vi "ABB Attendance report.vi"(10 "Report in":string) -> (2 "Report out":string)   [LabVIEW 2017]
uses:
  ABB global.vi
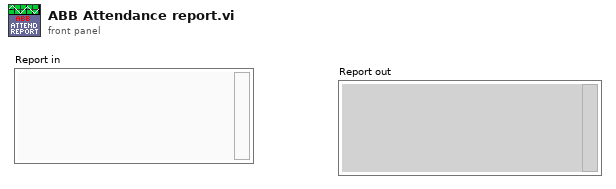
[diagram p1: front panel]
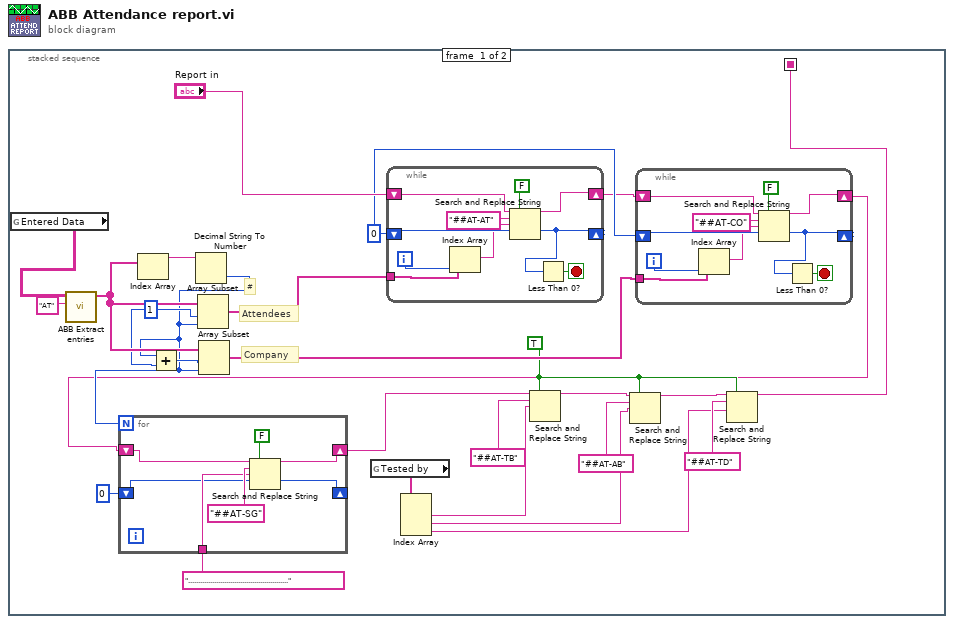
[diagram p0: block diagram]
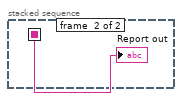
[diagram p2: hidden frame]
diagram:
  n1 = stacked-sequence {
    seq-local: [w14 _] -> [_ w55]
    frame #0 {
      w10 = TRUE ("replace all? (F)")
      w19 = 0
      w22 = 1 ("index")
      # "Company"
      # "Attendees"
      # "#"
      n2 = global read "ABB global.vi" "Entered Data"() -> (w24:string[][])
      n3 = call "ABB Extract entries.vi"("Entry ID"="AT", "Entry table in"=w24) -> ("Selected Entries"=w23:string[])  [unwired: 9 in]
      n4 = Index Array(array=w23) -> (element=w26:string)  [unwired: 1 in]
      n5 = Decimal String To Number(string=w26) -> (number=w5:i32)  [unwired: 2 in, 1 out]
      n6 = Add(x=w5, y=w22) -> (x+y=w21:i32)
      n7 = Array Subset(array=w23, index=w22, length=w5) -> (w20:string[])
      n8 = Array Subset(array=w23, index=w21, length=w5) -> (w17:string[])
      n9 = global read "ABB global.vi" "Tested by"() -> (w9:string[])
      n10 = while {
        shift-right: [w52] -> w18
        shift-left: "Report in" -> [w54]
        tunnel: w20 -> [w47]
        shift-right: [w48] -> _
        shift-left: w19 -> [w51]
        i -> [w46]
        stop <- w49 stop-if-true
        n11 = Index Array(array=w47, index=w46) -> (element=w45:string)
        n12 = Search and Replace String(replace all?=FALSE ("replace all? (F)"), input string=w54, search string="##AT-AT", replace string=w45, offset=w51) -> (result string=w52:string, offset past replacement=w48:i32)  [unwired: 3 in, 2 out]
        n13 = Less Than 0?(x=w48) -> (x < 0?=w49:bool)
      }
      n14 = Index Array(array=w9) -> (element #1=w8:string, element #2=w7:string, element #3=w6:string)  [unwired: 3 in]
      n15 = while {
        shift-right: [w42] -> w4
        shift-left: w18 -> [w44]
        tunnel: w17 -> [w37]
        shift-right: [w38] -> _
        shift-left: w19 -> [w41]
        i -> [w36]
        stop <- w39 stop-if-true
        n16 = Index Array(array=w37, index=w36) -> (element=w35:string)
        n17 = Search and Replace String(replace all?=FALSE ("replace all? (F)"), input string=w44, search string="##AT-CO", replace string=w35, offset=w41) -> (result string=w42:string, offset past replacement=w38:i32)  [unwired: 3 in, 2 out]
        n18 = Less Than 0?(x=w38) -> (x < 0?=w39:bool)
      }
      n19 = for {
        N: w5 -> [_]
        shift-right: [w30] -> w2
        shift-left: w4 -> [w31]
        tunnel: ".................................................." -> [w32]
        shift-right: [w28] -> _
        shift-left: 0 ("offset past replacement") -> [w29]
        n20 = Search and Replace String(replace all?=FALSE ("replace all? (F)"), input string=w31, search string="##AT-SG", replace string=w32, offset=w29) -> (result string=w30:string, offset past replacement=w28:i32)  [unwired: 3 in, 2 out]
      }
      n21 = Search and Replace String(replace all?=w10, input string=w2, search string="##AT-TB", replace string=w8) -> (result string=w16:string)  [unwired: 4 in, 3 out]
      n22 = Search and Replace String(replace all?=w10, input string=w16, search string="##AT-AB", replace string=w7) -> (result string=w15:string)  [unwired: 4 in, 3 out]
      n23 = Search and Replace String(replace all?=w10, input string=w15, search string="##AT-TD", replace string=w6) -> (result string=w14:string)  [unwired: 4 in, 3 out]
    }
    frame #1 {
      "Report out" <- w55
    }
  }
